vi "Uniform.vi"(0 "Input 3":u8[][](array[numeric]), 4 "bottom":i16, 5 "Input 2":u8[][](array[numeric]), 6 "right":i16, 7 "Input 1":u8[][](array[numeric]), 9 "seed in":i32=-1, 10 "samples":i32, 11 "Numeric":dbl) -> (1 "Output 3":u8[][](array[numeric]), 2 "Output 2":u8[][](array[numeric]), 3 "Output 1":u8[][](array[numeric]))   [LabVIEW 2016]
uses:
  <vilib>/Analysis/NI_AALBase.lvlib
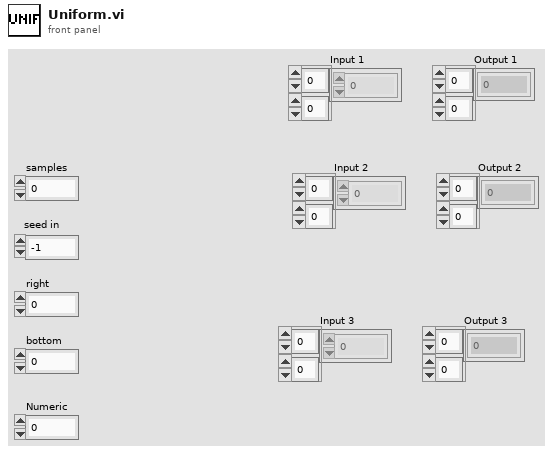
[diagram p1: front panel]
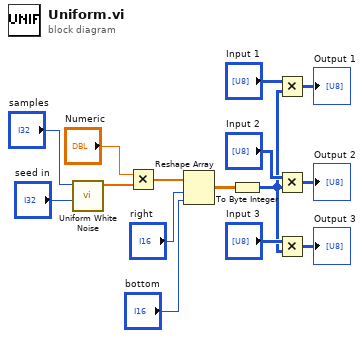
[diagram p0: block diagram]
diagram:
  n1 = call <vilib>:"Uniform White Noise.vi"("seed"="seed in", "samples"="samples") -> ("uniform white noise"=w8:dbl[])  [unwired: 8 in, 1 out]
  n2 = Multiply(x="Numeric", y=w8) -> (x*y=w12:dbl[])
  n3 = Reshape Array(w12, "right", "bottom") -> (w10:dbl[][])
  n4 = To Byte Integer(number=w10) -> (8bit integer=w1:i8[][])
  n5 = Multiply(x="Input 1", y=w1) -> (x*y=→"Output 1":u8[][])
  n6 = Multiply(x="Input 2", y=w1) -> (x*y=→"Output 2":u8[][])
  n7 = Multiply(x="Input 3", y=w1) -> (x*y=→"Output 3":u8[][])
